vi "Test Harness.vi"() -> ()   [LabVIEW 2020]
panel:
  out "All Words Found":bool
  out "Execution Time":dbl
  in  "Word List":string[](array[string])=["YELLOW", "ORANGE", "PURPLE", "BLUE", "GREEN", "RED"]
  in  "Word Search Grid":string[][](array[string])=[["R", "B", "L", "U", "E", "W"], ["E", "G", "N", "A", "R", "O"], ["D", "B", "C", "E", "W", "L"], ["L", "L", "D", "K", "V", "L"], ["P", "U", "R", "P", "L", "E"], ["N", "E", "E", "R", "G", "Y"]]
  # "Use this Test Harness VI to time your Word Search solution (and ensure it works correctly)."
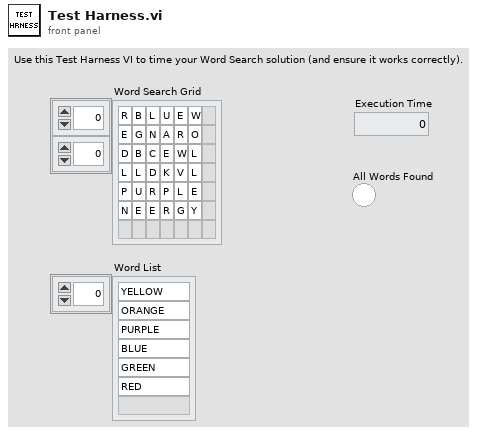
[diagram p1: front panel]
types:
  T1 = typedef "Solutions--map.ctl" = map{string, T2[]}
  T2 = typedef "Letter Index--cluster.ctl" = cluster{"Row":i32, "Column":i32}
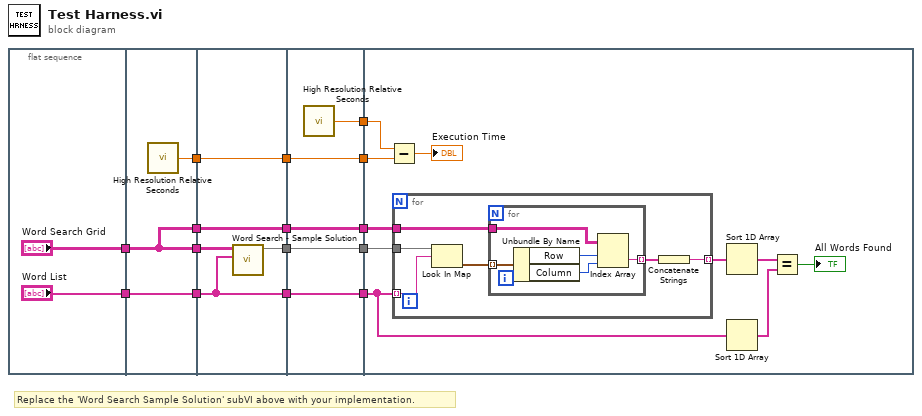
[diagram p0: block diagram]
diagram:
  # "Replace the 'Word Search Sample Solution' subVI above with your implementation."
  n1 = flat-sequence {
    tunnel: ["Word Search Grid"] -> w15
    tunnel: ["Word List"] -> w14
    tunnel: w15 -> [w18]
    tunnel: w14 -> [w20]
    tunnel: [w20] -> w13
    tunnel: [w18] -> w12
    tunnel: [w19] -> w8
    tunnel: [w18] -> w1
    tunnel: w13 -> [w22]
    tunnel: w12 -> [w25]
    tunnel: [w24] -> w11
    tunnel: w8 -> [w23]
    tunnel: [w23] -> w7
    tunnel: [w22] -> w4
    tunnel: [w21] -> w2
    tunnel: w1 -> [w21]
    tunnel: w11 -> [w30]
    tunnel: [w30] -> w10
    tunnel: [w29] -> w9
    tunnel: w7 -> [w28]
    tunnel: [w28] -> w6
    tunnel: [w27] -> w5
    tunnel: w4 -> [w27]
    tunnel: [w26] -> w3
    tunnel: w2 -> [w26]
    tunnel: w10 -> [w37]
    tunnel: w9 -> [w40]
    tunnel: w6 -> [w39]
    tunnel: w5 -> [w34]
    tunnel: w3 -> [w36]
    frame #0 {
    }
    frame #1 {
      n2 = call <vilib>:"High Resolution Relative Seconds.vi"() -> ("relative seconds"=w19:dbl)
    }
    frame #2 {
      n3 = call "Word Search - Sample Solution.vi"("Word List"=w22, "Word Search Grid"=w25) -> ("Solutions"=w24:T1)  [unwired: 9 in]
    }
    frame #3 {
      n4 = call <vilib>:"High Resolution Relative Seconds.vi"() -> ("relative seconds"=w29:dbl)
    }
    frame #4 {
      n5 = Subtract(x=w40, y=w39) -> (x-y=→"Execution Time":dbl)
      n6 = for {
        tunnel: w34 -> [w45] mode=indexing
        tunnel: w37 -> [w46]
        tunnel: w36 -> [w43]
        tunnel: [w41] -> w35 mode=indexing
        n7 = Look In Map(map=w46, key=w45) -> (value=w44:T2[])  [unwired: 1 in, 1 out]
        n8 = for {
          tunnel: w44 -> [w51] mode=indexing
          tunnel: w43 -> [w49]
          tunnel: [w47] -> w42 mode=indexing
          n9 = Unbundle By Name(w51) -> ("Row"=w50:i32, "Column"=w48:i32)
          n10 = Index Array(array=w49, index (row)=w50, index (col)=w48) -> (element=w47:string)
        }
        n11 = Concatenate Strings(w42) -> (w41:string)
      }
      n12 = Sort 1D Array(array=w35) -> (sorted array=w33:string[])
      n13 = Sort 1D Array(array=w34) -> (sorted array=w32:string[])
      n14 = Equal?(x=w33, y=w32) -> (x = y?=→"All Words Found":bool)
    }
  }
